vi "ReplacingNames.vi"() -> ()   [LabVIEW 2020]
panel:
  in  "Table Control":string[][](table)
  out "x = y?":bool
  out "subarray 2":string[](array[string])
  out "element":string
  out "subarray":string[][](array[string])
  out "index of element":i32
  out "Headers":string[][](array[string])
  in  "Path":path
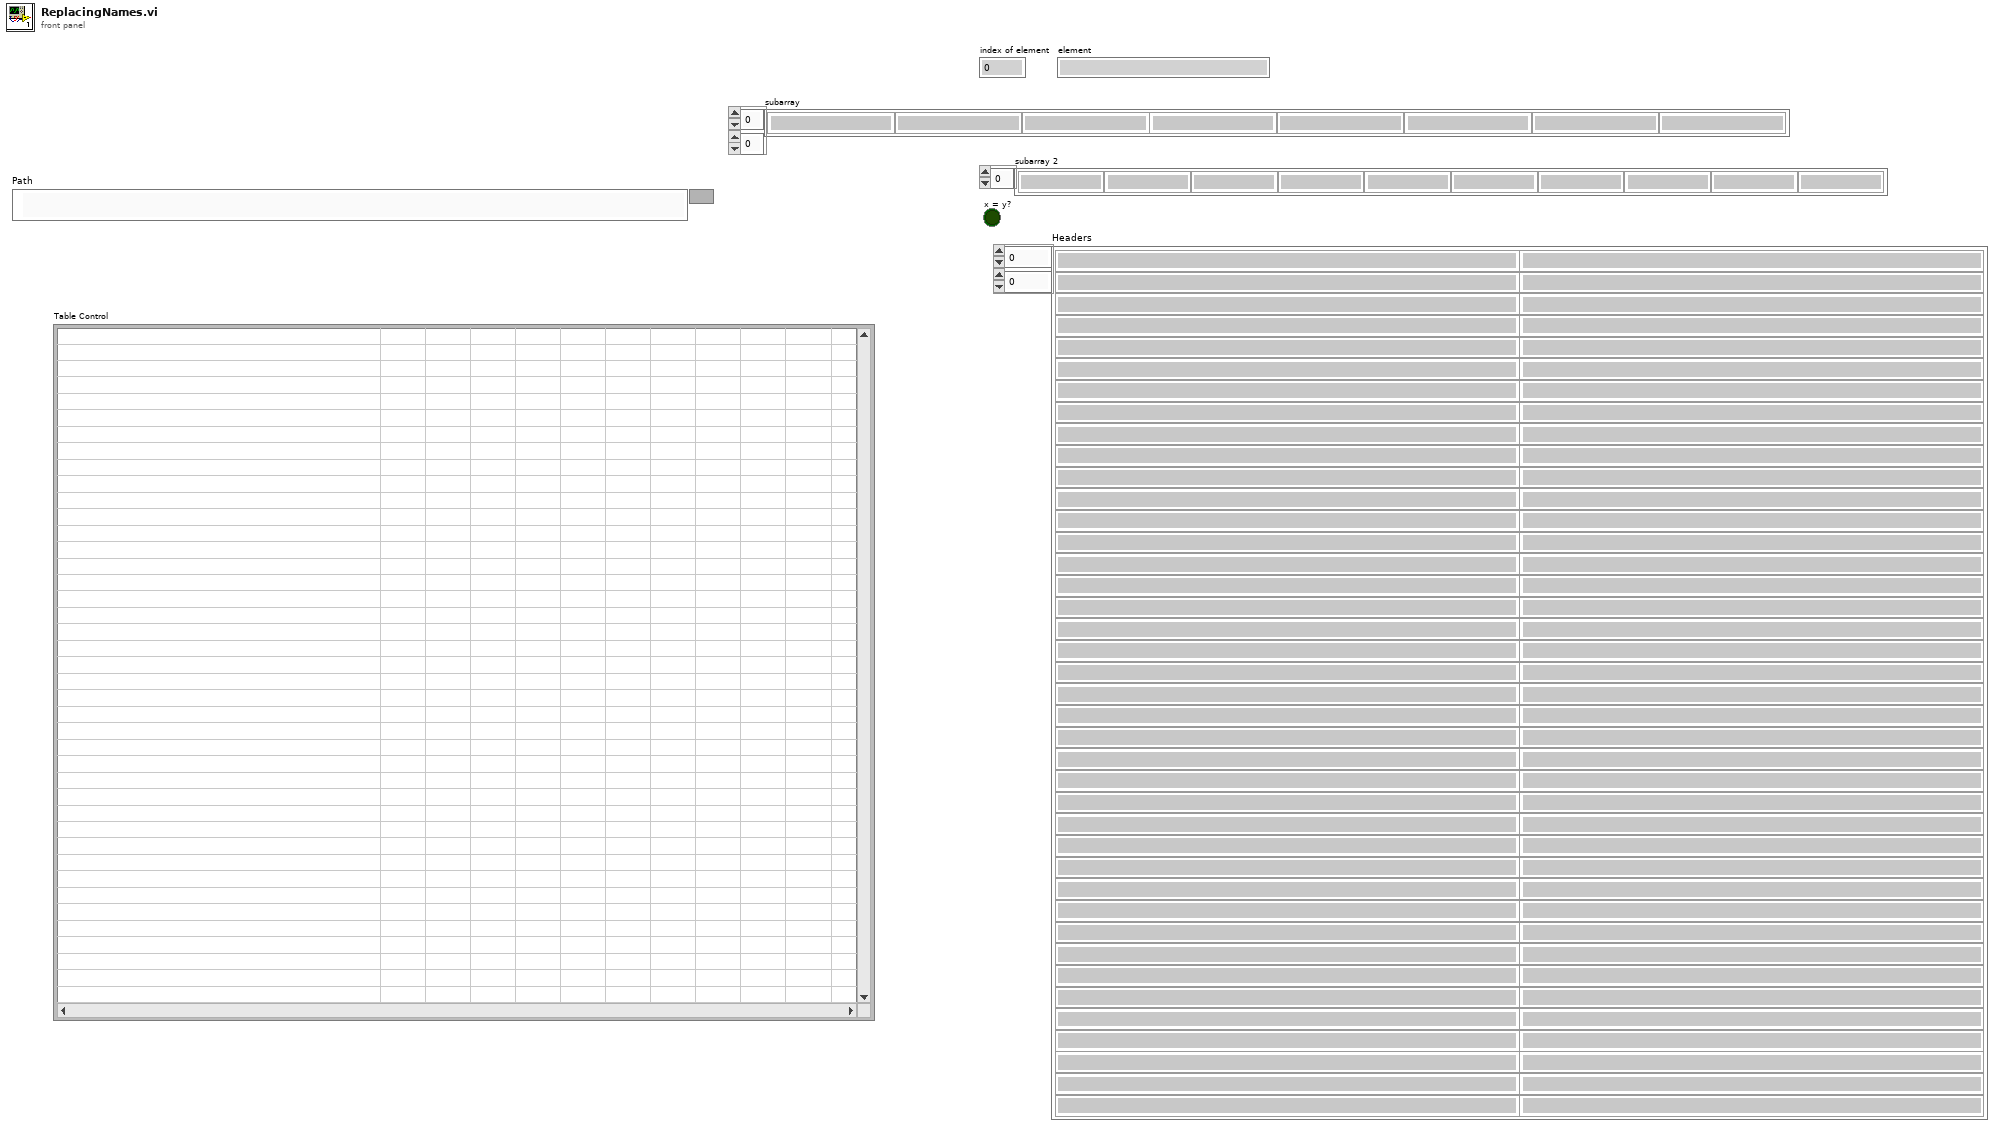
[diagram p1: front panel]
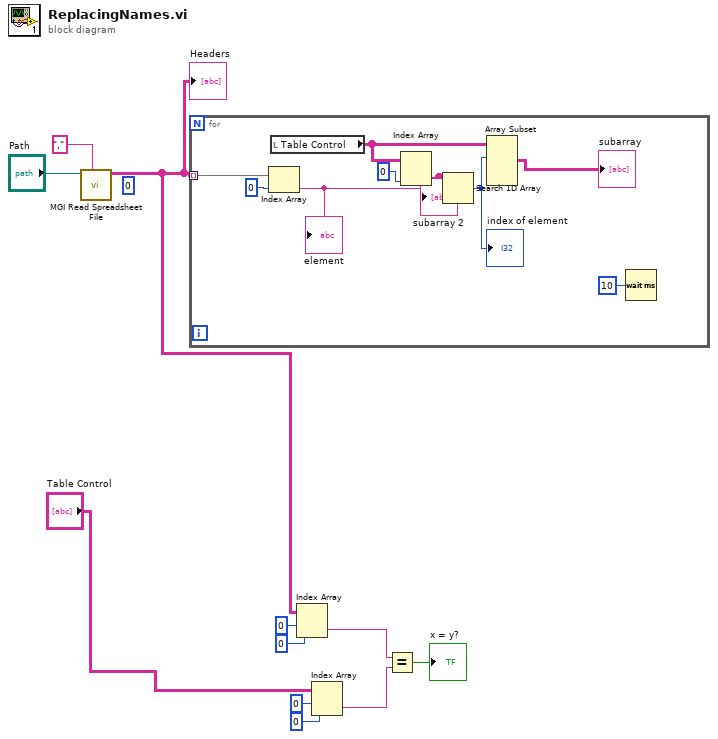
[diagram p0: block diagram]
diagram:
  (unwired) 0 ("index (row)")
  n1 = call <userlib>:"MGI Read Spreadsheet File.vi"("Delimiter (Tab)"=",", "Path"="Path") -> ("Headers"=w5:string[][])  [unwired: 5 in, 4 out]
  "Headers" <- w5
  n2 = for {
    tunnel: w5 -> [w20] mode=indexing
    n3 = Index Array(array=w20, index=0) -> (element=w18:string)
    "element" <- w18
    n4 = local read "Table Control"() -> (w15:string[][])
    n5 = Index Array(array=w15, index (col)=0 ("index")) -> (element=w16:string[])  [unwired: 1 in]
    "subarray 2" <- w16
    n6 = Search 1D Array(1D array=w16, element=w18) -> (index of element=w14:i32)  [unwired: 1 in]
    "index of element" <- w14
    n7 = Array Subset(array=w15, index (row)=w14) -> (→"subarray":string[][])  [unwired: 3 in]
    n8 = Wait (ms)(milliseconds to wait=u32 10) -> ()  [unwired: 1 out]
  }
  n9 = Index Array(array=w5, index (row)=0, index (col)=0 ("disabled index (col)")) -> (element=w4:string)
  n10 = Index Array(array="Table Control", index (row)=0, index (col)=0 ("disabled index (col)")) -> (element=w3:string)
  n11 = Equal?(x=w4, y=w3) -> (x = y?=→"x = y?":bool)
